vi "UpdateProjectFiles.vi"(11 "Command line args":string) -> (2 "Output":string, 3 "Error Code":i32)   [LabVIEW 2015, in "veristand-steps-build-tools.lvlib"]
uses:
  veristand-steps-build-tools.lvlib
panel:
  # "This VI is used to build the VeriStand Step Types manually or using an automated build system.\n\nThis VI performs the following actions:\n\n1. Reads the VeriStand Step Types version from the version file in the top level of the repository.\n\n2. Forms staging paths and creates new directories on disk if needed.\n\n3. Updates VeristandSteps.csproj file XML to use correct VeriStand and TestStand .NET assemblies\n\n4. Builds the VeriStandSteps.dll assembly using MSBuild\n\n5. Updates NI_VeristandTypes.ini file XML to new Step Types version\n\n6. Places all built files in appropriate staging directories from step (2)\n\n7. Places documentaion/tutorial files to staging directories created in step (2)."
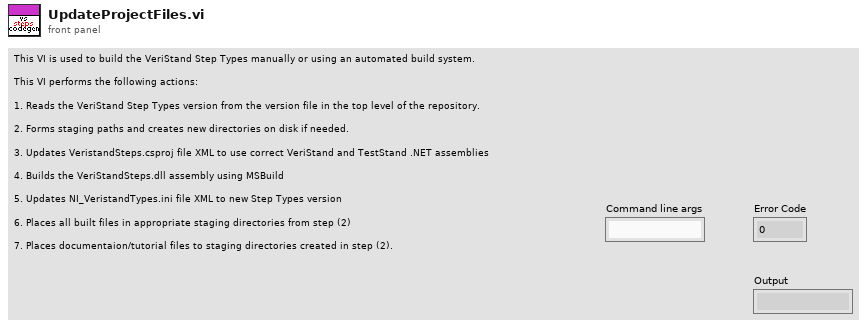
[diagram p1: front panel]
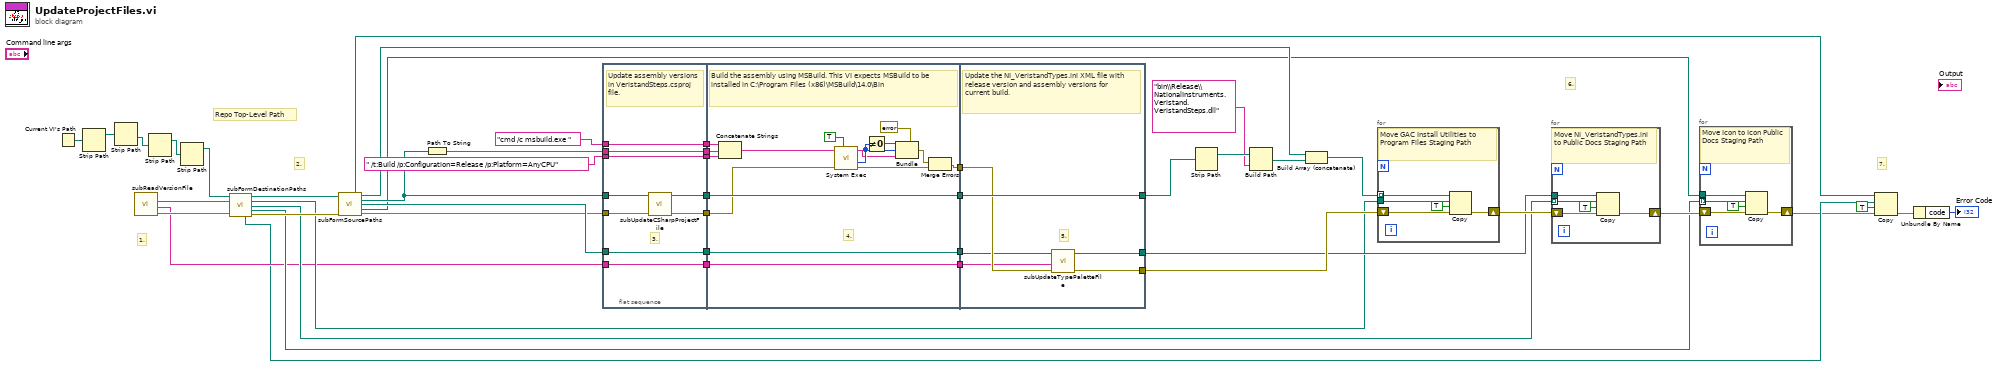
[diagram p0: block diagram]
diagram:
  # "7."
  # "Repo Top-Level Path"
  # "6."
  # "2."
  # "1."
  n1 = Current VI's Path() -> (path=w12:path)
  n2 = Strip Path(path=w12) -> (stripped path=w13:path)  [unwired: 1 out]
  n3 = Strip Path(path=w13) -> (stripped path=w14:path)  [unwired: 1 out]
  n4 = call "subReadVersionFile.vi"() -> ("error out"=w16:errorcluster, "Step Types Version"=w9:string, "TestStand Versions"=w8:string)  [unwired: 9 in]
  n5 = Strip Path(path=w14) -> (stripped path=w15:path)  [unwired: 1 out]
  n6 = Strip Path(path=w15) -> (stripped path=w11:path)  [unwired: 1 out]
  n7 = call "subFormDestinationPaths.vi"("Repo Top-Level Path"=w11, "TestStand Version String"=w8, "error in"=w16) -> ("Repo Top-Level Path out"=w10:path, "Program Files Destination Path"=w19:path, "TypePalettes Paths"=w17:path[], "Icon Paths"=w18:path[], "VS Steps Pub Docs Path"=w5:path, "error out"=w20:errorcluster)  [unwired: 7 in]
  n8 = call "subFormSourcePaths.vi"("Repo Top-level"=w10, "error in (no error)"=w20) -> ("Documentation Source Path"=w6:path, "GACUtilityPaths"=w24:path[], "CSharp Assembly Project Path"=w23:path, "TypePalette File Path"=w22:path, "Icon File Path"=w7:path, "error out"=w21:errorcluster)  [unwired: 8 in]
  n9 = Path To String(path=w23) -> (string=w32:string)
  n10 = flat-sequence {
    tunnel: " /t:Build /p:Configuration=Release /p:Platform=AnyCPU" ("string") -> [w55]
    tunnel: "cmd /c msbuild.exe " -> [w56]
    tunnel: [w56] -> w44
    tunnel: [w55] -> w43
    tunnel: w23 -> [w54]
    tunnel: [w53] -> w42
    tunnel: [w52] -> w41
    tunnel: w32 -> [w51]
    tunnel: [w51] -> w31
    tunnel: w22 -> [w50]
    tunnel: [w50] -> w29
    tunnel: w9 -> [w49]
    tunnel: [w49] -> w28
    tunnel: w21 -> [w48]
    tunnel: [w72] -> w39
    tunnel: w41 -> [w72]
    tunnel: w42 -> [w67]
    tunnel: w43 -> [w69]
    tunnel: w44 -> [w70]
    tunnel: [w58] -> w38
    tunnel: w31 -> [w66]
    tunnel: [w65] -> w30
    tunnel: w29 -> [w65]
    tunnel: w28 -> [w64]
    tunnel: [w64] -> w27
    tunnel: [w78] -> w25
    tunnel: w39 -> [w78]
    tunnel: [w77] -> w37
    tunnel: w38 -> [w76]
    tunnel: w30 -> [w74]
    tunnel: w27 -> [w75]
    tunnel: [w73] -> w26
    frame #0 {
      # "3."
      # "Update assembly versions in VeristandSteps.csproj file."
      n11 = call "subUpdateCSharpProjectFile.vi"("error in (no error)"=w48, ".csproj path"=w54) -> ("error out"=w53:errorcluster, ".csproj path out"=w52:path)  [unwired: 8 in]
    }
    frame #1 {
      # "4."
      # "Build the assembly using MSBuild. This VI expects MSBuild to be installed in C:\\Program Files (x86)\\MSBuild\\14.0\\Bin"
      n12 = Concatenate Strings(w70, w66, w69) -> (w68:string)
      n13 = call <vilib>:"System Exec.vi"("wait until completion? (T)"=TRUE, "error in (no error)"=w67, "command line"=w68) -> ("error out"=w59:errorcluster, "return code"=w62:i32, "standard output"=w57:string)  [unwired: 5 in, 1 out]
      n14 = Not Equal To 0?(x=w62) -> (x != 0?=w61:bool)
      n15 = Bundle(cluster=errorcluster {"status"=FALSE, "code"=0, "source"=""} ("error constant"), "status"=w61, "code"=w62, "source"=w57) -> (w60:errorcluster)
      n16 = Merge Errors(w60, w59) -> (w58:errorcluster)
    }
    frame #2 {
      # "5."
      # "Update the NI_VeristandTypes.ini XML file with release version and assembly versions for current build."
      n17 = call "subUpdateTypePaletteFile.vi"("error in (no error)"=w76, "Step Types Version"=w75, "TypePalette .ini file location"=w74) -> ("error out"=w77:errorcluster, "Type Palettes File Path out"=w73:path)  [unwired: 7 in]
    }
  }
  n18 = Strip Path(path=w25) -> (stripped path=w46:path)  [unwired: 1 out]
  n19 = Build Path(base path=w46, name or relative path="bin\\Release\\NationalInstruments.Veristand.VeristandSteps.dll") -> (appended path=w36:path)
  n20 = Build Array (concatenate)(w24, w36) -> (w35:path[])
  n21 = for {
    shift-right: [w83] -> w34
    shift-left: w37 -> [w82]
    tunnel: w35 -> [w81] mode=indexing
    tunnel: w19 -> [w80]
    # "Move GAC Install Utilities to Program Files Staging Path"
    n22 = Copy(8:w82, 9:TRUE ("overwrite (F)"), 10:w80, 11:w81) -> (0:w83:errorcluster)  [unwired: 1 in, 2 out]
  }
  n23 = for {
    shift-right: [w88] -> w33
    shift-left: w34 -> [w87]
    tunnel: w26 -> [w85]
    tunnel: w17 -> [w84] mode=indexing
    # "Move NI_VeristandTypes.ini to Public Docs Staging Path"
    n24 = Copy(8:w87, 9:TRUE ("overwrite (F)"), 10:w84, 11:w85) -> (0:w88:errorcluster)  [unwired: 1 in, 2 out]
  }
  n25 = for {
    shift-right: [w93] -> w4
    shift-left: w33 -> [w92]
    tunnel: w18 -> [w90] mode=indexing
    tunnel: w7 -> [w89]
    # "Move Icon to Icon Public Docs Staging Path"
    n26 = Copy(8:w92, 9:TRUE ("overwrite (F)"), 10:w90, 11:w89) -> (0:w93:errorcluster)  [unwired: 1 in, 2 out]
  }
  n27 = Copy(8:w4, 9:TRUE ("overwrite (F)"), 10:w5, 11:w6) -> (0:w2:errorcluster)  [unwired: 1 in, 2 out]
  n28 = Unbundle By Name(w2) -> ("code"=→"Error Code":i32)
